vi "Initialize Resistor Interface.vi"(8 "error in (no error)":errorcluster, 10 "Enum Refnum":refnum<vi>[](array[refnum]), 11 "Color Box Refnum":refnum<vi>[](array[refnum])) -> (0 "error out":errorcluster)   [LabVIEW 2018, in "Front Panel Interface.lvlib"]
doc: "Initializes the resistor Front Panel interface to a known state.\n\nThe VI receives the arrays of <b>Enum Refnums</b> and <b>Color Box Refnums</b> corresponding to the six resistor band selectors and six resistor band ColorBox controls.\n\nIt sets the <b>Visible</b> property of all band selectors and ColorBox controls to <b>TRUE</b>, making all six resistor bands and their corresponding selectors visible.\n\nThis VI only establishes the initial Front Panel visibility state. It does not configure the interface according to the selected number of bands."
uses:
  Front Panel Interface.lvlib
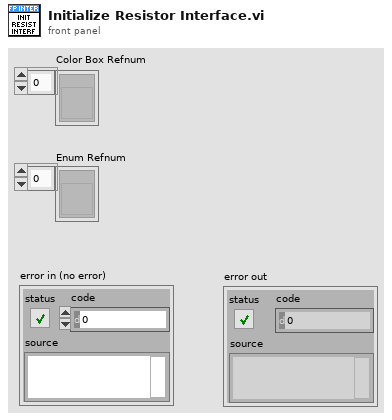
[diagram p1: front panel]
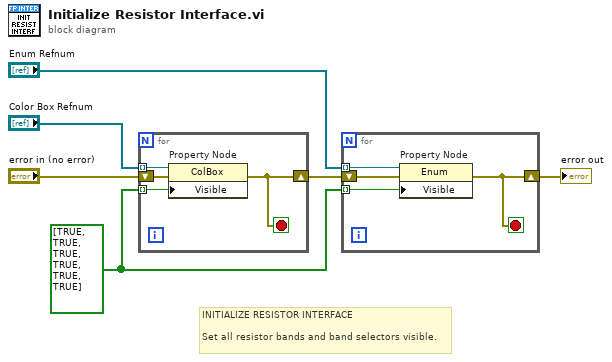
[diagram p0: block diagram]
diagram:
  w1 = bool[] [TRUE, TRUE, TRUE, TRUE, TRUE, TRUE]
  # "INITIALIZE RESISTOR INTERFACE\n\nSet all resistor bands and band selectors visible."
  n1 = for {
    tunnel: "Color Box Refnum" -> [w10] mode=indexing
    tunnel: w1 -> [w9] mode=indexing
    shift-right: [w7] -> w4
    shift-left: "error in (no error)" -> [w8]
    stop <- w7 stop-if-true
    n2 = property on="Property Node" class="ColBox"(reference=w10, error in=w8, "Visible"=w9) -> (error out=w7:errorcluster)  [unwired: 1 out]
  }
  n3 = for {
    tunnel: w1 -> [w11] mode=indexing
    shift-right: [w13] -> w2
    shift-left: w4 -> [w14]
    tunnel: "Enum Refnum" -> [w12] mode=indexing
    stop <- w13 stop-if-true
    n4 = property on="Property Node" class="Enum"(reference=w12, error in=w14, "Visible"=w11) -> (error out=w13:errorcluster)  [unwired: 1 out]
  }
  "error out" <- w2
